vi "Top Main.vi"   [LabVIEW 2020]
uses:
  User Event/FGV Action.ctl
  User Event/User Event.lvlib
  Module/Configuration DB/DB.lvlib
  Module/Control/Control.lvlib
  Module/Display Console/Display.lvlib
  Module/Error/Error.lvlib
  Module/Sensor/Sensor.lvlib
  Module/User Console/User Console.lvlib
types:
  T1 = typedef "User Event.lvlib/FGV Action.ctl" = enum16{"Create", "Get", "Destroy"}
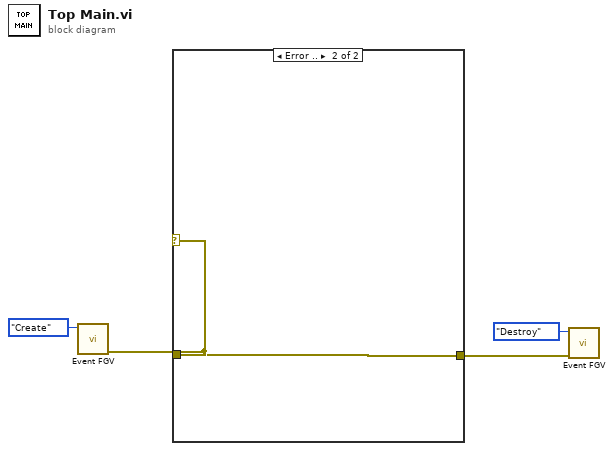
[diagram p0: block diagram]
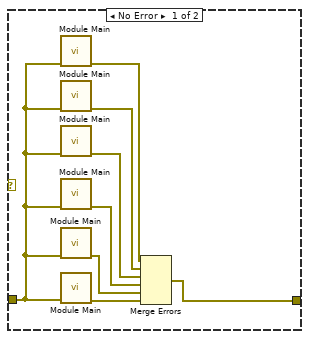
[diagram p2: hidden frame]
diagram:
  n1 = call "Event FGV.vi"("FGV Action"=FGV_Action."Create") -> ("error out"=w2:errorcluster)  [unwired: 9 in, 1 out]
  n2 = case shown="Error .." w2 {
    tunnel: w2 -> [w12 w13]
    tunnel: [w5 w13] -> w1
    frame No Error {
      n3 = call "Module Main.vi"("error in (no error)"=w12) -> ("error out"=w11:errorcluster)  [unwired: 10 in]
      n4 = call "Module Main.vi"("error in (no error)"=w12) -> ("error out"=w10:errorcluster)  [unwired: 10 in]
      n5 = call "Module Main.vi"("error in (no error)"=w12) -> ("error out"=w9:errorcluster)  [unwired: 10 in]
      n6 = call "Module Main.vi"("error in (no error)"=w12) -> ("error out"=w8:errorcluster)  [unwired: 10 in]
      n7 = call "Module Main.vi"("error in (no error)"=w12) -> ("error out"=w7:errorcluster)  [unwired: 10 in]
      n8 = call "Module Main.vi"("error in (no error)"=w12) -> ("error out"=w6:errorcluster)  [unwired: 10 in]
      n9 = Merge Errors(w11, w10, w9, w8, w7, w6) -> (w5:errorcluster)
    }
    frame Error {
    }
  }
  n10 = call "Event FGV.vi"("error in (no error)"=w1, "FGV Action"=FGV_Action."Destroy") -> ()  [unwired: 8 in, 2 out]
